vi "test.ingest_video.vi"   [LabVIEW 2020]
uses:
  datasources/source/create_s3.vi
  datasources/source/source.lvclass
  datasources/dataset/dataset.lvclass
  81c5314d-0c17-4e40-9591-806fc92e59be.vi
  Nominal Client/Nominal Client.lvclass
  40e2c779-94f0-4ff6-913c-6196809b7e71.vi
  nominal types/timestampManifest/timestampManifest.lvlib
  nominal types/timestampManifest/create.mcap_id.vi
  nominal types/timestampManifest/create.noManifest_trueFrameRate.vi
  nominal types/timestampManifest/create.s3path.vi
  nominal types/timestampManifest/create.noManifest_scale_factor.vi
  nominal types/timestampManifest/create.noManifest_endingTimestamp.vi
  nominal types/timestampManifest/create.mcap_topic.vi
  datasources/target/target.lvclass
  datasources/target/create_from_existing.vi
  datasources/source/create_gcs.vi
  datasources/target/create_new.vi
  nominal types/channelConfig/channelConfig.lvclass
  Nominal Client/ingest_video.vi
  nominal types/properties/properties.lvclass
  nominal types/timestampManifest/mcap/mcap.lvclass
  C:/code/labview-client/lv_src/nominal types/timestampManifest/timestampManifest/timestampManifest.lvclass
  C:/code/labview-client/lv_src/Nominal Client/datasources/payload/payload.lvclass
  C:/code/labview-client/lv_src/nominal types/timestampManifest/mcap/mcap.lvclass
  nominal types/timestampManifest/noManifest/noManifest.lvclass
  C:/code/labview-client/lv_src/nominal types/timestampManifest/noManifest/noManifest.lvclass
  nominal types/timestampManifest/s3path/s3path.lvclass
  C:/code/labview-client/lv_src/nominal types/timestampManifest/s3path/s3path.lvclass
  datasources/s3/s3.lvclass
  C:/code/labview-client/lv_src/Nominal Client/datasources/source/source.lvclass
  C:/code/labview-client/lv_src/Nominal Client/datasources/s3/s3.lvclass
  datasources/gcs/gcs.lvclass
  C:/code/labview-client/lv_src/Nominal Client/datasources/gcs/gcs.lvclass
types:
  T1 = cluster{"dataset":refnum<class "dataset.lvclass">, "channelConfig":refnum<class "channelConfig.lvclass">}
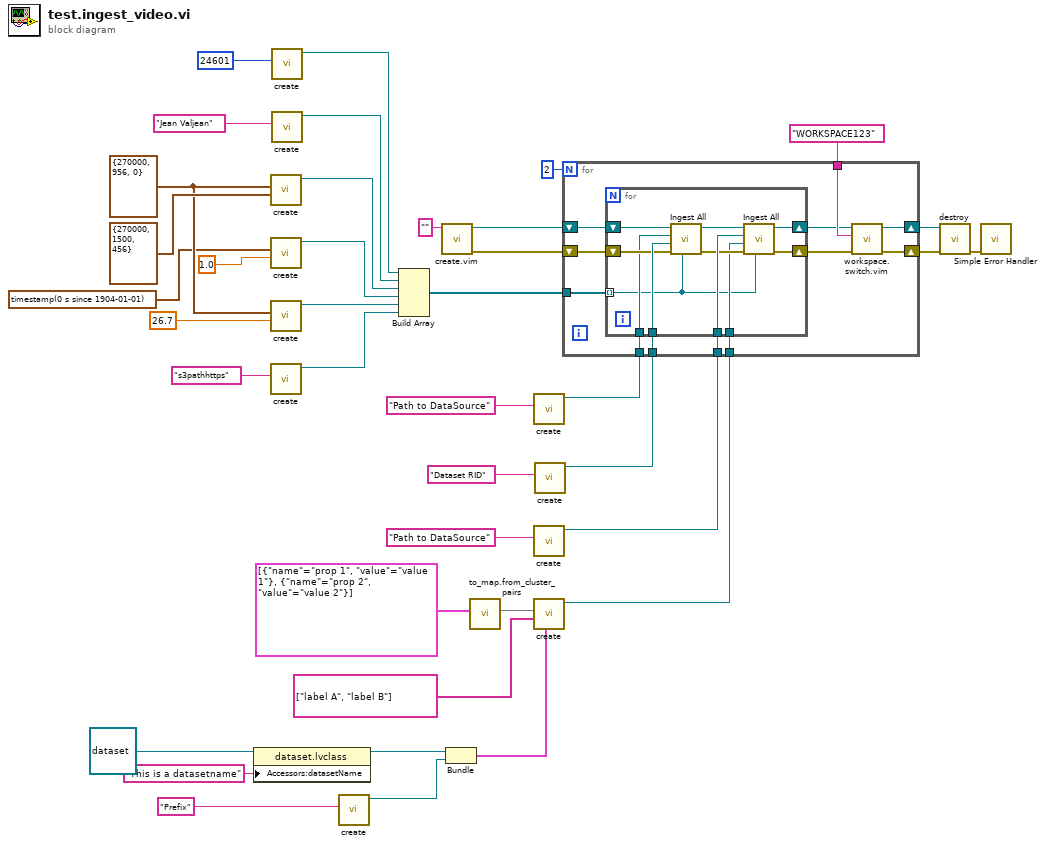
[diagram p0: block diagram]
diagram:
  w5 = cluster{"seconds":i64, "nanos":i64, "picos":i64} {"seconds"=270000, "nanos"=956, "picos"=0} ("startingTimestamp")
  n1 = property class="dataset.lvclass"(reference=refnum<class "dataset.lvclass"> refnum ("dataset"), "Accessors:datasetName"="This is a datasetname" ("datasetName")) -> (reference out=w31:refnum<class "dataset.lvclass">)  [unwired: 1 in, 1 out]
  n2 = call-poly "create.vi"("endingTimestamp"=cluster{"seconds":i64, "nanos":i64, "picos":i64} {"seconds"=270000, "nanos"=1500, "picos"=456}, "startingTimestamp"=w5) -> ("Timestamp Manifest"=w26:refnum<class "noManifest.lvclass">)  [unwired: 9 in]
  n3 = call-poly "create.vi"("scaleFactor"=1.0, "startingTimestamp"=timestamp(0 s since 1904-01-01)) -> ("Timestamp Manifest"=w25:refnum<class "noManifest.lvclass">)  [unwired: 9 in]
  n4 = call-poly "create.vi"("trueFrameRate"=26.7, "startingTimestamp"=w5) -> ("Timestamp Manifest"=w24:refnum<class "noManifest.lvclass">)  [unwired: 9 in]
  n5 = call-poly "create.vi"("path"="s3pathhttps") -> ("Timestamp Manifest"=w23:refnum<class "s3path.lvclass">)  [unwired: 10 in]
  n6 = call-poly "create.vi"("id"=24601) -> ("Timestamp Manifest"=w28:refnum<class "mcap.lvclass">)  [unwired: 10 in]
  n7 = call-poly "create.vi"("topic"="Jean Valjean") -> ("Timestamp Manifest"=w27:refnum<class "mcap.lvclass">)  [unwired: 10 in]
  n8 = call "create.vi"("prefixTreeDelimiter"="Prefix") -> ("channelConfig"=w6:refnum<class "channelConfig.lvclass">)  [unwired: 10 in]
  n9 = Build Array(w28, w27, w26, w25, w24, w23) -> (w22:refnum<class "timestampManifest.lvclass">[])
  n10 = call "create.vim"("API Token (string or path)"="") -> ("error out"=w35:errorcluster, "Nominal Client"=w36:refnum<class "Nominal Client.lvclass">)  [unwired: 9 in]
  n11 = Bundle("dataset"=w31, "channelConfig"=w6) -> (w9:T1)  [unwired: 1 in]
  n12 = call "to_map.from_cluster_pairs.vi"("properties (cluster pairs)"=cluster{"name":string, "value":string}[] [{"name"="prop 1", "value"="value 1"}, {"name"="prop 2", "value"="value 2"}] ("properties")) -> ("properties (map)"=w1:map{string, string})  [unwired: 10 in]
  n13 = call-poly "create.vi"("Path"="Path to DataSource") -> ("source"=w14:refnum<class "s3.lvclass">)  [unwired: 10 in]
  n14 = call-poly "create.vi"("Path"="Path to DataSource") -> ("source"=w10:refnum<class "gcs.lvclass">)  [unwired: 10 in]
  n15 = call-poly "create.vi"("Optional"=w9, "Labels"=string[] ["label A", "label B"] ("labels"), "Properties"=w1) -> ("New Target"=w8:refnum<class "target.lvclass">)  [unwired: 8 in]
  n16 = call-poly "create.vi"("dataset RID"="Dataset RID" ("RID")) -> ("Existing Target"=w12:refnum<class "target.lvclass">)  [unwired: 10 in]
  n17 = for {
    N: 2 -> [_]
    tunnel: w12 -> [w51]
    tunnel: w14 -> [w44]
    tunnel: w10 -> [w50]
    tunnel: w8 -> [w43]
    shift-right: [w47] -> w37
    shift-left: w35 -> [w49]
    shift-right: [w46] -> w39
    shift-left: w36 -> [w48]
    tunnel: "WORKSPACE123" ("RID") -> [w45]
    tunnel: w22 -> [w40]
    n18 = for {
      tunnel: w51 -> [w62]
      tunnel: w50 -> [w61]
      tunnel: w44 -> [w56]
      tunnel: w43 -> [w55]
      shift-right: [w53] -> w41
      shift-left: w49 -> [w58]
      shift-right: [w54] -> w42
      shift-left: w48 -> [w57]
      tunnel: w40 -> [w52] mode=indexing
      n19 = call-poly "Ingest All.vi"("Timestamp Manifest"=w52, "error in"=w58, "Target"=w62, "Source"=w56, "Nominal Client in"=w57) -> ("error out"=w59:errorcluster, "Nominal Client out"=w60:refnum<class "Nominal Client.lvclass">)  [unwired: 3 in, 2 out]
      n20 = call-poly "Ingest All.vi"("Timestamp Manifest"=w52, "error in"=w59, "Target"=w55, "Source"=w61, "Nominal Client in"=w60) -> ("error out"=w53:errorcluster, "Nominal Client out"=w54:refnum<class "Nominal Client.lvclass">)  [unwired: 3 in, 2 out]
    }
    n21 = call "workspace.switch.vim"("error in"=w41, "Workspace RID (string or path)"=w45, "Nominal Client in"=w42) -> ("error out"=w47:errorcluster, "Nominal Client out"=w46:refnum<class "Nominal Client.lvclass">)  [unwired: 7 in]
  }
  n22 = call "destroy.vi"("error in"=w37, "Nominal Client"=w39) -> ("error out"=w29:errorcluster)  [unwired: 9 in]
  n23 = call <vilib>:"Simple Error Handler.vi"("error in (no error)"=w29) -> ()  [unwired: 4 in, 5 out]
